vi "Initialize.vi"(8 "error in (no error)":errorcluster, 10 "Microscope Configuration":T1={"Serial Port"="COM2", "Microscope Type"=enum."TE2000", "Detection Settings"=[]}, 11 "Microscope In":refnum<class "Microscope.lvclass">) -> (0 "error out":errorcluster, 3 "Microscope out":refnum<class "Microscope.lvclass">)   [LabVIEW 2023, in "Microscope.lvlib" / "Microscope.lvclass"]
uses:
  Microscope.lvclass
  Resources/Type Defs/Microscope Configuration.ctl
  Resources/Type Defs/Microscope Type.ctl
  Microscope.lvclass/Microscope.ctl
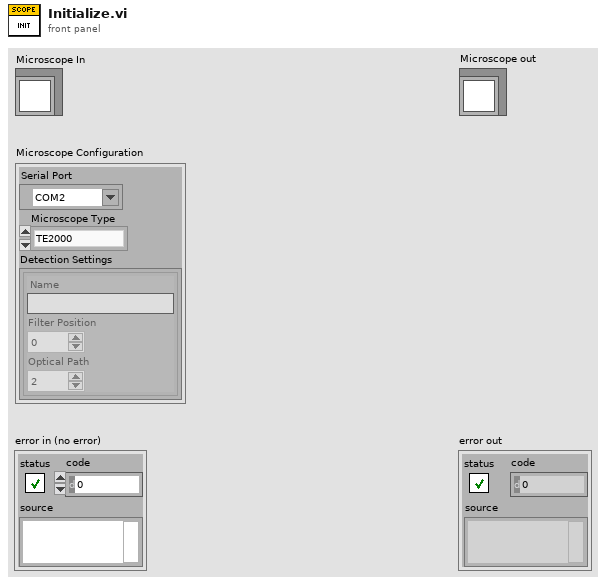
[diagram p1: front panel]
types:
  T1 = typedef "Microscope Configuration.ctl" = cluster{"Serial Port":refnum<visa-resource-name>, "Microscope Type":T2, "Detection Settings":cluster{"Name":string, "Filter Position":u16, "Optical Path":u16}[]}
  T2 = typedef "Microscope Type.ctl" = enum16{"Disable", "TE2000", "Eclipse Ti", "Ti2"}
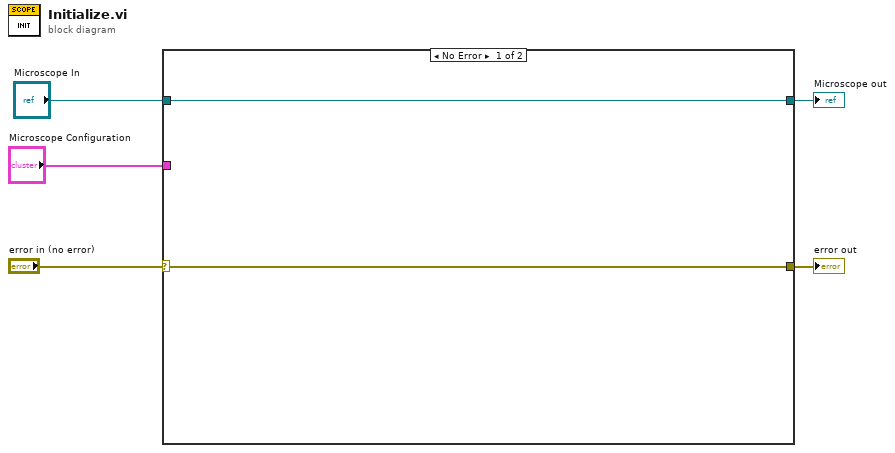
[diagram p0: block diagram]
diagram:
  n1 = case shown="No Error" "error in (no error)" {
    selector: "error in (no error)" -> [w6 w9]
    tunnel: [w6 w9] -> w5
    tunnel: "Microscope In" -> [w7 w8]
    tunnel: [w7 w8] -> w2
    tunnel: "Microscope Configuration" -> [_ _]
    frame No Error {
    }
    frame Error {
    }
  }
  "error out" <- w5
  "Microscope out" <- w2
